vi "RunTimeExitApp.vi"(8 "error in (no error)":errorcluster) -> (0 "error out":errorcluster)   [LabVIEW 2015]
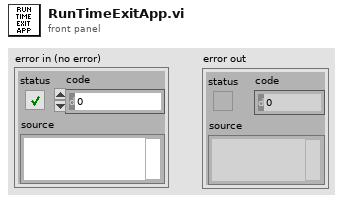
[diagram p1: front panel]
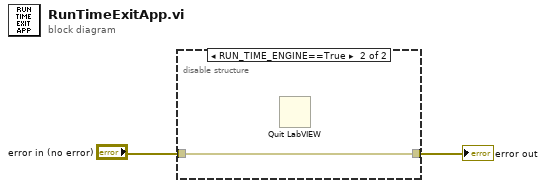
[diagram p0: block diagram]
diagram:
  n1 = disable-structure "Conditional Disable Structure" shown="RUN_TIME_ENGINE==True" {
    disable-tunnel: "error in (no error)" -> [w3 w4]
    disable-tunnel: [w3 w4] -> w2
    frame condition #0 (active) {
    }
    frame condition #1 {
      n2 = Quit LabVIEW() -> ()  [unwired: 1 in]
    }
  }
  "error out" <- w2
